vi "RL.vi"(8 "Size (m)":cluster{"Width":sgl, "Height":sgl}={"Width"=nan, "Height"=nan} caption="Size (m) (NaN=no change)" {"Height" format="%.2p"; "Width" format="%.2p"}, 9 "Center coordinates (m)":cluster{"Xc":sgl, "Yc":sgl}={"Xc"=nan, "Yc"=nan} caption="Center coordinates (m) (NaN=no change)" {"Yc" format="%.2p"; "Xc" format="%.2p"}, 10 "XYData":sgl[][](array[numeric]) format="%#_5p", 11 "Application ref in":refnum<vi>) -> (0 "rollout":dbl[](array[numeric]), 1 "Boolean":bool, 2 "Data":sgl[][](array[numeric]) format="%#_5p", 3 "Application ref out":refnum<vi>)   [LabVIEW 2020]
uses:
  <userlib>/Nanonis Prog Interface V5/Nanonis Prog Interface.lvlib
panel:
  in  "Python version":string="3.6"
  in  "module path":path=path "C:/Users/e0321251/Documents/GitHub/PyNanois/labview/Tip.py"
  in  "Python version 4":string="3.6"
  in  "module path 4":path=path "C:/Users/e0321251/Documents/GitHub/PyNanois/labview/RL.py"
  in  "array":dbl[](array[numeric])=[1.0, 2.0]
  out "Error out":errorcluster
  in  "error in (no error)":errorcluster
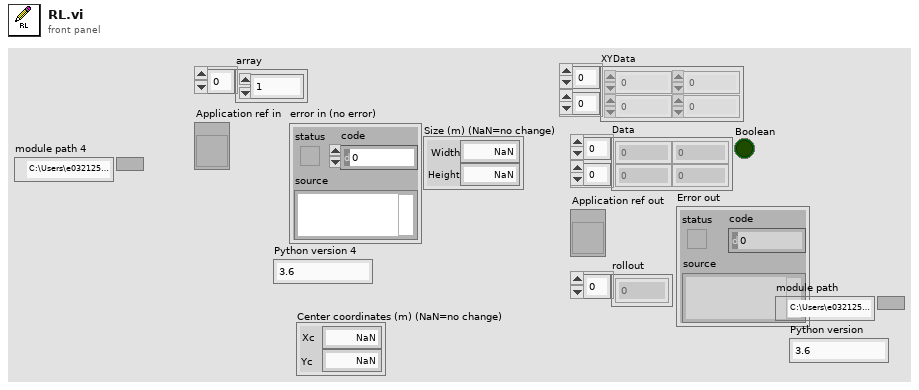
[diagram p1: front panel]
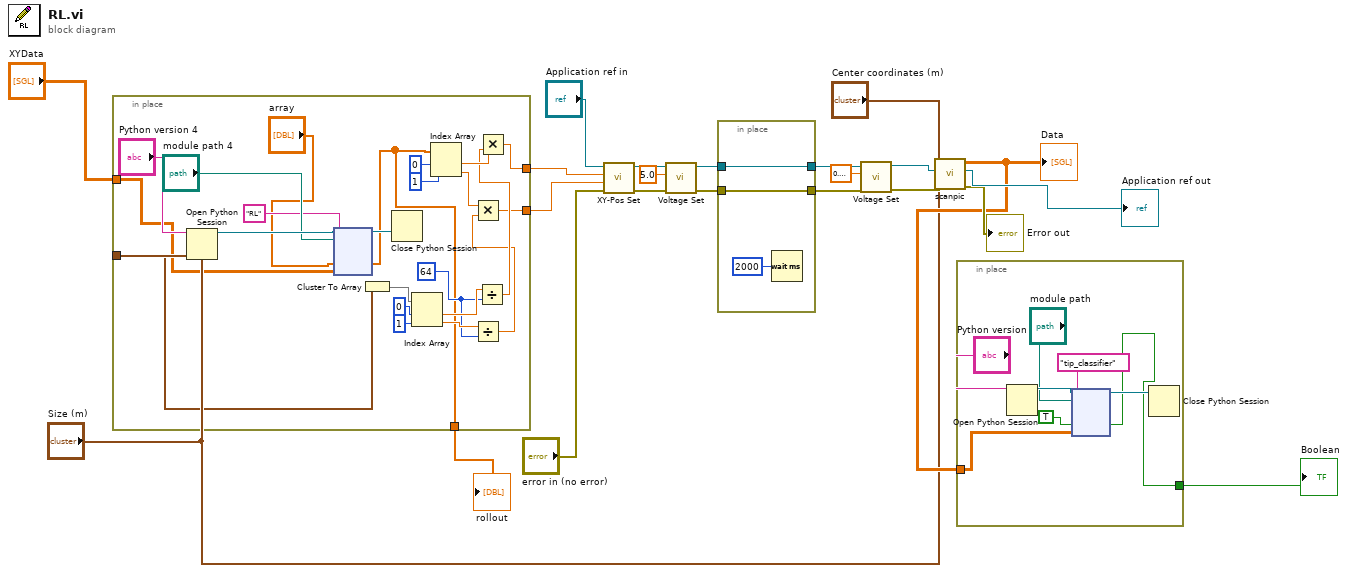
[diagram p0: block diagram]
diagram:
  n1 = in-place {
    in-place-border: "XYData" -> [w24]
    in-place-border: "Size (m)" -> [w40]
    in-place-border: [w32] -> w4
    in-place-border: [w31] -> w3
    in-place-border: [w23] -> w1
    w37 = 64
    n2 = Open Python Session(python version="Python version 4") -> (session out=w30:refnum<k35>)  [unwired: 2 in, 1 out]
    n3 = node(w30, "module path 4", "RL" ("function name"), "array", w24) -> (w29:refnum<k35>, w23:dbl[])  [unwired: 2 in, 3 out]
    n4 = Cluster To Array(cluster=w40) -> (array=w41:sgl[])
    n5 = Close Python Session(session in=w29) -> ()  [unwired: 1 in, 1 out]
    n6 = Index Array(array=w41, index #1=0 ("index"), index #2=1 ("index")) -> (element #1=w39:sgl, element #2=w38:sgl)
    n7 = Index Array(array=w23, index #1=0 ("index"), index #2=1 ("index")) -> (element #1=w36:dbl, element #2=w34:dbl)
    n8 = Divide(x=w38, y=w37) -> (x/y=w33:sgl)
    n9 = Multiply(x=w34, y=w33) -> (x*y=w31:dbl)
    n10 = Divide(x=w39, y=w37) -> (x/y=w35:sgl)
    n11 = Multiply(x=w36, y=w35) -> (x*y=w32:dbl)
  }
  "rollout" <- w1
  n12 = call <userlib>:"XY-Pos Set.vi"("error in (no error)"="error in (no error)", "Y (m)"=w3, "X (m)"=w4, "Application ref in"="Application ref in") -> ("error out"=w17:errorcluster, "Application ref out"=w19:refnum<vi>)  [unwired: 4 in]
  n13 = call <userlib>:"Voltage Set.vi"("Error in (no error)"=w17, "Bias (V)"=sgl 5.0, "Application ref in"=w19) -> ("Error out"=w15:errorcluster, "Application ref out"=w16:refnum<vi>)  [unwired: 7 in]
  n14 = in-place {
    in-place-border: w16 -> [w47]
    in-place-border: w15 -> [w48]
    in-place-border: [w48] -> w13
    in-place-border: [w47] -> w14
    n15 = Wait (ms)(milliseconds to wait=u32 2000) -> ()  [unwired: 1 out]
  }
  n16 = call <userlib>:"Voltage Set.vi"("Error in (no error)"=w13, "Bias (V)"=sgl 0.1, "Application ref in"=w14) -> ("Error out"=w10:errorcluster, "Application ref out"=w11:refnum<vi>)  [unwired: 7 in]
  n17 = call "scanpic.vi"("error in (no error)"=w10, "Size (m)"="Size (m)", "Application ref in"=w11, "Center coordinates (m)"="Center coordinates (m)") -> ("Error out"=→"Error out":errorcluster, "Application ref out"=→"Application ref out":refnum<vi>, "Data"=w6:sgl[][])  [unwired: 5 in]
  "Data" <- w6
  n18 = in-place {
    in-place-border: w6 -> [w50]
    in-place-border: [w49] -> w2
    n19 = Open Python Session(python version="Python version") -> (session out=w56:refnum<k35>)  [unwired: 2 in, 1 out]
    n20 = node(w56, "module path", "tip_classifier" ("function name"), TRUE, w50) -> (w55:refnum<k35>, w49:bool)  [unwired: 2 in, 3 out]
    n21 = Close Python Session(session in=w55) -> ()  [unwired: 1 in, 1 out]
  }
  "Boolean" <- w2
